vi "Read Test.vi"(8 "error in (no error)":errorcluster, 9 "data table":T1, 10 "data dictionary":refnum<class "data dictionary.lvclass">, 11 "runtime in":refnum<class "SystemLink runtime.lvclass">) -> (0 "error out":errorcluster, 2 "Pass":bool[](array[boolean]), 3 "runtime out":refnum<class "SystemLink runtime.lvclass">)   [LabVIEW 2015, in "SystemLink Tag Module tests.lvlib"]
uses:
  SystemLink Tag Module tests.lvlib
  module/execution/SystemLink runtime.lvclass
  <vilib>/NI/Tag Bus/table/data table.ctl
  <vilib>/NI/Tag Bus/dictionary/data dictionary.lvclass
  <vilib>/Skyline/Tag/Shared/typedefs/DataType.ctl
  <vilib>/NI/Tag Bus/dictionary/data dictionary.lvclass/data dictionary.ctl
  <vilib>/NI/Tag Bus/dictionary/lookup polymorphs/locate double.vi
  <vilib>/NI/Tag Bus/table/data polymorphs/read one/read Double.vi
  <vilib>/NI/Tag Bus/dictionary/lookup polymorphs/locate I32.vi
  <vilib>/NI/Tag Bus/table/data polymorphs/read one/read I32.vi
  <vilib>/NI/Tag Bus/dictionary/lookup polymorphs/locate String.vi
  <vilib>/NI/Tag Bus/table/data polymorphs/read one/read String.vi
  <vilib>/NI/Tag Bus/dictionary/lookup polymorphs/locate U64.vi
  <vilib>/NI/Tag Bus/table/data polymorphs/read one/read U64.vi
  <vilib>/NI/Tag Bus/dictionary/lookup polymorphs/locate Boolean.vi
  <vilib>/NI/Tag Bus/table/data polymorphs/read one/read Boolean.vi
  <vilib>/NI/Tag Bus/dictionary/search/find data index.vi
  <vilib>/NI/Tag Bus/dictionary/search/search string list.vi
  <vilib>/NI/Tag Bus/dictionary/tag not found.vi
  <vilib>/Skyline/Tag/Wrapper/Wrapper AMQP_class/Open Tag AMQP.vi
  <vilib>/Skyline/Tag/Wrapper/Wrapper_class/Write Tag (Boolean).vi
  <vilib>/Skyline/Tag/Wrapper/Wrapper_class/Close Tag (Single).vi
  <vilib>/Skyline/Tag/Wrapper/Wrapper_class/Write Tag (U64).vi
  <vilib>/Skyline/Tag/Wrapper/Wrapper_class/Write Tag (DBL).vi
  <vilib>/Skyline/Tag/Wrapper/Wrapper_class/Write Tag (I32).vi
  <vilib>/Skyline/Tag/Wrapper/Wrapper_class/Write Tag (String).vi
  <vilib>/NI/Tag Bus/table/data table.lvlib
  <vilib>/Skyline/Tag/Wrapper/Wrapper_class/NI Skyline Tag.lvclass
  <vilib>/Skyline/Tag/Wrapper/Wrapper AMQP_class/NI Skyline Tag AMQP.lvclass
  <vilib>/Skyline/Tag/Shared/NI Skyline Tag.lvlib
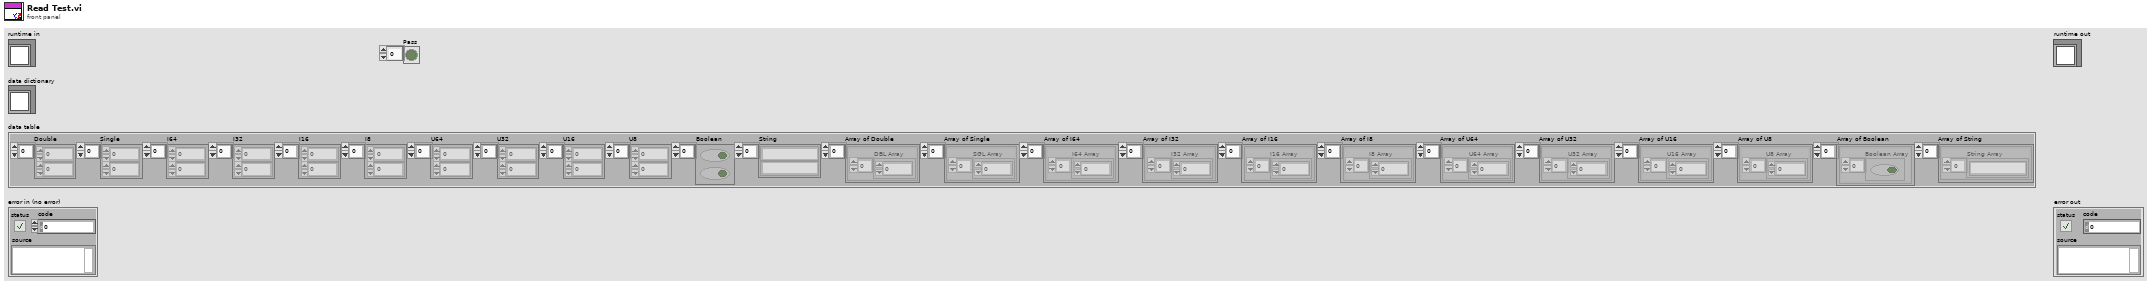
[diagram p1: front panel]
types:
  T1 = typedef "tag bus.lvlib/data table.lvlib/data table.ctl" = cluster{"Double":dbl[], "Single":sgl[], "I64":i64[], "I32":i32[], "I16":i16[], "I8":i8[], "U64":u64[], "U32":u32[], "U16":u16[], "U8":u8[], "Boolean":bool[], "String":string[], "Array of Double":cluster{"DBL Array":dbl[]}[], "Array of Single":cluster{"SGL Array":sgl[]}[], "Array of I64":cluster{"I64 Array":i64[]}[], "Array of I32":cluster{"I32 Array":i32[]}[], "Array of I16":cluster{"I16 Array":i16[]}[], "Array of I8":cluster{"I8 Array":i8[]}[], "Array of U64":cluster{"U64 Array":u64[]}[], "Array of U32":cluster{"U32 Array":u32[]}[], "Array of U16":cluster{"U16 Array":u16[]}[], "Array of U8":cluster{"U8 Array":u8[]}[], "Array of Boolean":cluster{"Boolean Array":bool[]}[], "Array of String":cluster{"String Array":string[]}[]}
  T2 = typedef "NI Skyline Tag.lvlib/DataType.ctl" = enum32{"Double", "I32", "String", "Boolean", "U64", "Timestamp"}
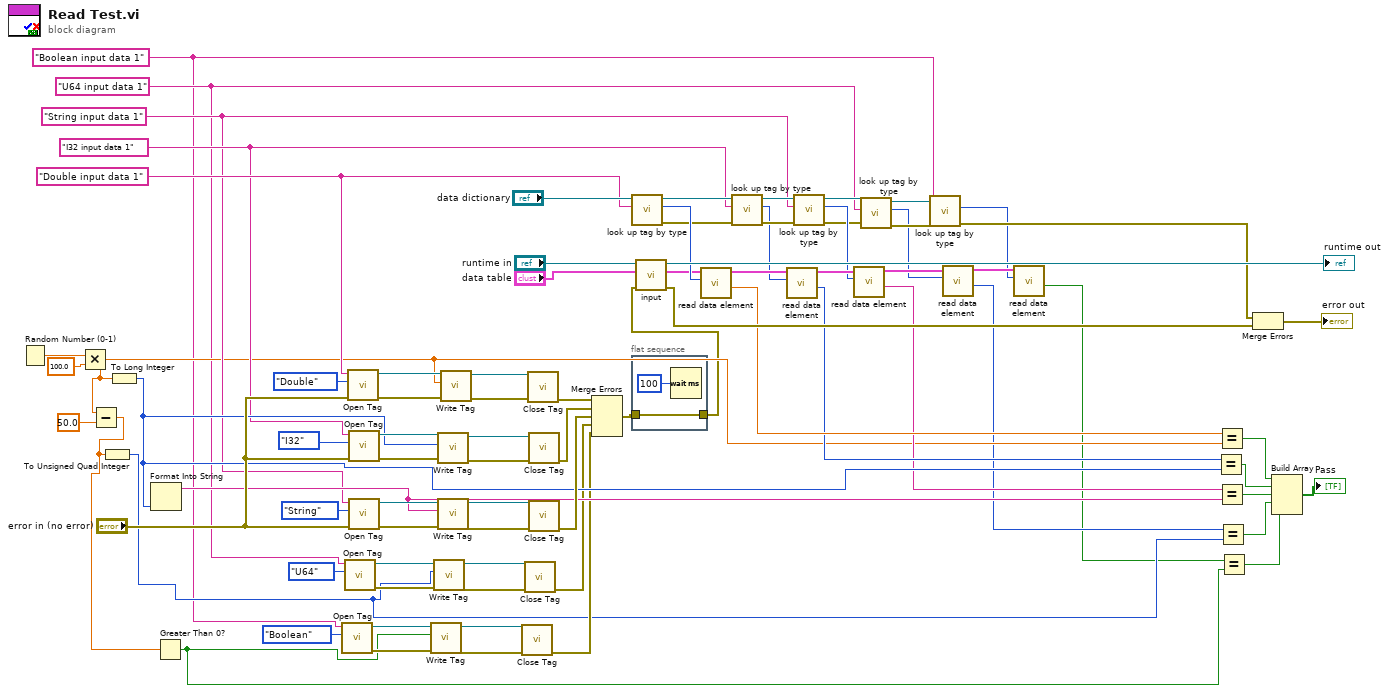
[diagram p0: block diagram]
diagram:
  w4 = "U64 input data 1" ("channel name")
  w3 = "Boolean input data 1" ("channel name")
  w37 = "String input data 1" ("channel name")
  w38 = "I32 input data 1" ("channel name")
  w39 = "Double input data 1" ("channel name")
  n1 = Random Number (0-1)() -> (number: 0 to 1=w53:dbl)
  n2 = Multiply(x=w53, y=100.0) -> (x*y=w25:dbl)
  n3 = Subtract(x=w25, y=50.0) -> (x-y=w23:dbl)
  n4 = To Unsigned Quad Integer(1:w23) -> (0:w18:u64)
  n5 = To Long Integer(number=w25) -> (32bit integer=w44:i32)
  n6 = Format Into String(w44) -> (resulting string=w43:string)  [unwired: 3 in, 1 out]
  n7 = Greater Than 0?(x=w23) -> (x > 0?=w17:bool)
  n8 = call-poly <vilib>:"Open Tag.vi"("data type"=DataType."Boolean", "path"=w3) -> ("error out"=w26:errorcluster, "tag out"=w29:refnum<class "NI Skyline Tag.lvclass">)  [unwired: 8 in]
  n9 = call-poly <vilib>:"Open Tag.vi"("data type"=DataType."U64", "path"=w4) -> ("error out"=w35:errorcluster, "tag out"=w32:refnum<class "NI Skyline Tag.lvclass">)  [unwired: 8 in]
  n10 = call-poly <vilib>:"Open Tag.vi"("error in (no error)"="error in (no error)", "data type"=DataType."Double", "path"=w39) -> ("error out"=w56:errorcluster, "tag out"=w66:refnum<class "NI Skyline Tag.lvclass">)  [unwired: 7 in]
  n11 = call-poly <vilib>:"Open Tag.vi"("error in (no error)"="error in (no error)", "data type"=DataType."I32", "path"=w38) -> ("error out"=w58:errorcluster, "tag out"=w65:refnum<class "NI Skyline Tag.lvclass">)  [unwired: 7 in]
  n12 = call-poly <vilib>:"Open Tag.vi"("error in (no error)"="error in (no error)", "data type"=DataType."String", "path"=w37) -> ("error out"=w59:errorcluster, "tag out"=w64:refnum<class "NI Skyline Tag.lvclass">)  [unwired: 7 in]
  n13 = call-poly <vilib>:"Write Tag.vi"("error in (no error)"=w26, "value"=w17, "tag in"=w29) -> ("error out"=w27:errorcluster, "tag out"=w28:refnum<class "NI Skyline Tag.lvclass">)  [unwired: 7 in]
  n14 = call-poly <vilib>:"Write Tag.vi"("error in (no error)"=w35, "value"=w18, "tag in"=w32) -> ("error out"=w34:errorcluster, "tag out"=w33:refnum<class "NI Skyline Tag.lvclass">)  [unwired: 7 in]
  n15 = call-poly <vilib>:"Write Tag.vi"("error in (no error)"=w58, "value"=w44, "tag in"=w65) -> ("error out"=w57:errorcluster, "tag out"=w62:refnum<class "NI Skyline Tag.lvclass">)  [unwired: 7 in]
  n16 = call-poly <vilib>:"Write Tag.vi"("error in (no error)"=w59, "value"=w43, "tag in"=w64) -> ("error out"=w60:errorcluster, "tag out"=w61:refnum<class "NI Skyline Tag.lvclass">)  [unwired: 7 in]
  n17 = call-poly <vilib>:"Write Tag.vi"("error in (no error)"=w56, "value"=w25, "tag in"=w66) -> ("error out"=w55:errorcluster, "tag out"=w63:refnum<class "NI Skyline Tag.lvclass">)  [unwired: 7 in]
  n18 = call-poly <vilib>:"Close Tag.vi"("error in (no error)"=w27, "tag in"=w28) -> ("error out"=w21:errorcluster)  [unwired: 9 in]
  n19 = call-poly <vilib>:"Close Tag.vi"("error in (no error)"=w34, "tag in"=w33) -> ("error out"=w22:errorcluster)  [unwired: 9 in]
  n20 = call-poly <vilib>:"Close Tag.vi"("error in (no error)"=w55, "tag in"=w63) -> ("error out"=w51:errorcluster)  [unwired: 9 in]
  n21 = call-poly <vilib>:"Close Tag.vi"("error in (no error)"=w57, "tag in"=w62) -> ("error out"=w50:errorcluster)  [unwired: 9 in]
  n22 = call-poly <vilib>:"Close Tag.vi"("error in (no error)"=w60, "tag in"=w61) -> ("error out"=w49:errorcluster)  [unwired: 9 in]
  n23 = Merge Errors(w51, w50, w49, w22, w21) -> (w1:errorcluster)
  n24 = call-poly <vilib>:"look up tag by type.vi"("name"=w39, "data dictionary in"="data dictionary") -> ("error out"=w73:errorcluster, "index"=w81:i32, "data dictionary out"=w72:refnum<class "data dictionary.lvclass">)  [unwired: 7 in]
  n25 = flat-sequence {
    tunnel: [w84] -> w2
    tunnel: w1 -> [w84]
    frame #0 {
      n26 = Wait (ms)(milliseconds to wait=u32 100) -> ()  [unwired: 1 out]
    }
  }
  n27 = call-dynamic "input.vi"("error in"=w2, "data table in"="data table", "SystemLin Tag Module runtime in"="runtime in") -> ("error out"=w82:errorcluster, "data table out"=w80:T1, "SystemLin Tag Module runtime out"=→"runtime out":refnum<class "SystemLink runtime.lvclass">)  [unwired: 6 in]
  n28 = call-poly <vilib>:"read data element.vi"("index"=w81, "data table in"=w80) -> ("value"=w42:dbl, "data table out"=w77:T1)  [unwired: 8 in]
  n29 = call-poly <vilib>:"look up tag by type.vi"("error in"=w73, "name"=w38, "data dictionary in"=w72) -> ("error out"=w74:errorcluster, "index"=w70:i32, "data dictionary out"=w71:refnum<class "data dictionary.lvclass">)  [unwired: 6 in]
  n30 = call-poly <vilib>:"read data element.vi"("index"=w70, "data table in"=w77) -> ("value"=w41:i32, "data table out"=w76:T1)  [unwired: 8 in]
  n31 = call-poly <vilib>:"look up tag by type.vi"("error in"=w74, "name"=w37, "data dictionary in"=w71) -> ("error out"=w15:errorcluster, "index"=w75:i32, "data dictionary out"=w16:refnum<class "data dictionary.lvclass">)  [unwired: 6 in]
  n32 = call-poly <vilib>:"read data element.vi"("index"=w75, "data table in"=w76) -> ("value"=w40:string, "data table out"=w10:T1)  [unwired: 8 in]
  n33 = call-poly <vilib>:"look up tag by type.vi"("error in"=w15, "name"=w4, "data dictionary in"=w16) -> ("error out"=w14:errorcluster, "index"=w8:i32, "data dictionary out"=w13:refnum<class "data dictionary.lvclass">)  [unwired: 6 in]
  n34 = call-poly <vilib>:"look up tag by type.vi"("error in"=w14, "name"=w3, "data dictionary in"=w13) -> ("error out"=w11:errorcluster, "index"=w7:i32)  [unwired: 6 in, 1 out]
  n35 = call-poly <vilib>:"read data element.vi"("index"=w8, "data table in"=w10) -> ("value"=w6:u64, "data table out"=w9:T1)  [unwired: 8 in]
  n36 = call-poly <vilib>:"read data element.vi"("index"=w7, "data table in"=w9) -> ("value"=w5:bool)  [unwired: 8 in, 1 out]
  n37 = Equal?(x=w41, y=w44) -> (x = y?=w47:bool)
  n38 = Equal?(x=w42, y=w25) -> (x = y?=w48:bool)
  n39 = Equal?(x=w40, y=w43) -> (x = y?=w46:bool)
  n40 = Equal?(x=w6, y=w18) -> (x = y?=w20:bool)
  n41 = Equal?(x=w5, y=w17) -> (x = y?=w19:bool)
  n42 = Merge Errors(w11, w82) -> (→"error out":errorcluster)
  n43 = Build Array(w48, w47, w46, w20, w19) -> (→"Pass":bool[])
